vi "PSD fitting.vi"(6 "DNA length (µm)":dbl=0.658, 8 "fsampling (Hz)":dbl=2800.0, 9 "Fit settings":T2={"#PSD Averages"=40, "Correct camera acquisition artifacts"=TRUE, "Autorange"=TRUE, "fstart (Hz)"=0.0, "Pendulum geometry"=FALSE, "Fit model"=FALSE} {"#PSD Averages" min=1}, 10 "X/Y data":dbl[](array[numeric])) -> (2 "Fit Results":T1, 3 "Power spectrum (um^2/Hz)":cluster{dbl[], "Spectrum out":dbl[]}[](graph))   [LabVIEW 2017]
uses:
  <vilib>/Analysis/NI_AALPro.lvlib
  <vilib>/Analysis/NI_AALBase.lvlib
panel:
  out "df (Hz)":dbl=0.18404907975460122 format="%.2f"
  # "Fit parameters"
  # "Calculated quantities"
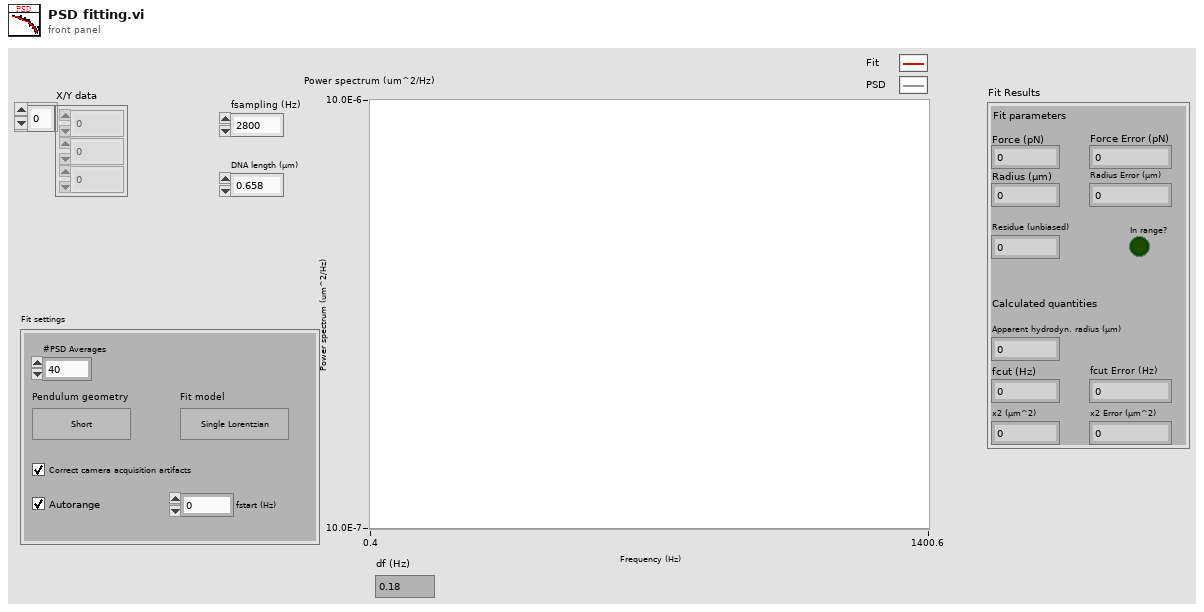
[diagram p1: front panel]
types:
  T1 = cluster{"fcut (Hz)":dbl, "x2 (µm^2)":dbl, "Force (pN)":dbl, "Radius (µm)":dbl, "Apparent hydrodyn. radius (µm)":dbl, "fcut Error (Hz)":dbl, "x2 Error (µm^2)":dbl, "Force Error (pN)":dbl, "Radius Error (µm)":dbl, "Residue (unbiased)":dbl, "In range?":bool}
  T2 = cluster{"#PSD Averages":u8, "Correct camera acquisition artifacts":bool, "Autorange":bool, "fstart (Hz)":dbl, "Pendulum geometry":bool, "Fit model":bool}
  T3 = cluster{"mean":dbl, "MSD (µm^2)":dbl, "RMS (µm)":dbl, "fc analytic (Hz)":dbl, "x2 analytic (Hz)":dbl, "RMS analytic (µm)":dbl, "F analytic (pN)":dbl, "fc fit (Hz)":dbl, "x2 fit (µm^2)":dbl, "RMS fit (µm)":dbl, "F fit (pN)":dbl, "R fit (µm)":dbl, "Rhydro (µm)":dbl, "fc Error (Hz)":dbl, "x2fit Error (µm^2)":dbl, "RMSfit Error (µm)":dbl, "Ffit Error (pN)":dbl, "Rfit Error (µm)":dbl, "correlation":dbl, "residue":dbl}
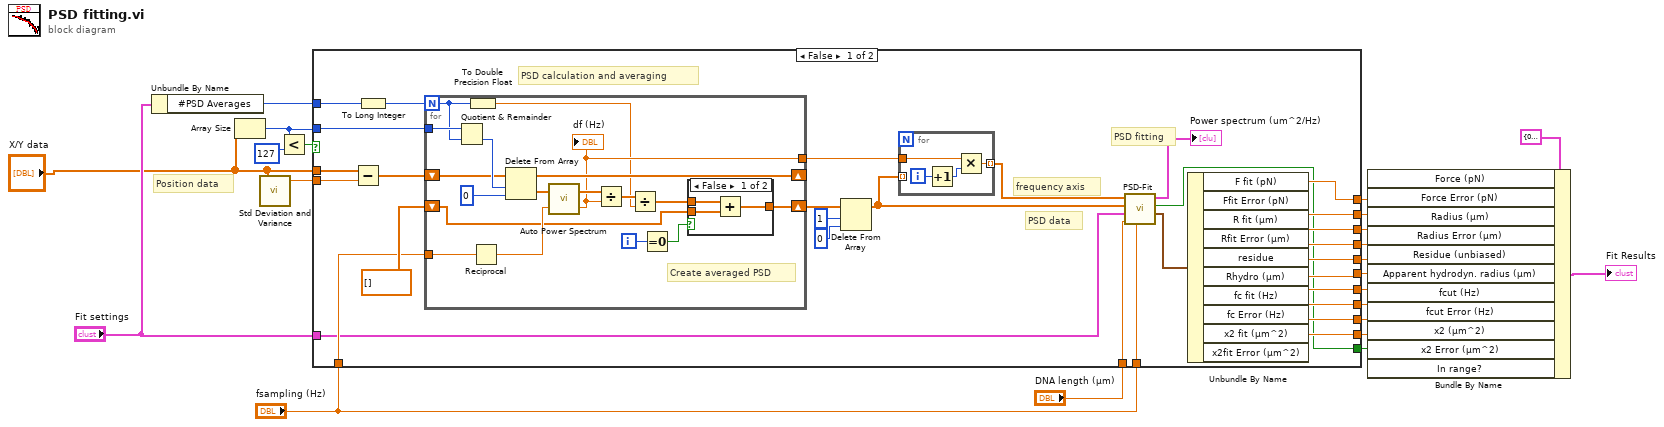
[diagram p0: block diagram]
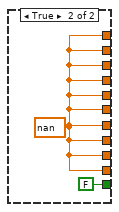
[diagram p3: hidden frame]
diagram:
  # "Position data"
  n1 = Unbundle By Name("Fit settings") -> ("#PSD Averages"=w19:u8)
  n2 = Array Size(array="X/Y data") -> (size(s)=w20:i32)
  n3 = call <vilib>:"Std Deviation and Variance.vi"("X"="X/Y data") -> ("mean"=w17:dbl)  [unwired: 1 in, 2 out]
  n4 = Less?(x=w20, y=127) -> (x < y?=w21:bool)
  n5 = case shown="False" w21 {
    tunnel: "X/Y data" -> [w50 _]
    tunnel: [w52 w80] -> w10
    tunnel: [w30 w80] -> w9
    tunnel: w20 -> [w51 _]
    tunnel: [w46 w80] -> w8
    tunnel: [w29 w80] -> w7
    tunnel: [w45 w80] -> w6
    tunnel: [w44 w80] -> w5
    tunnel: [w43 w80] -> w13
    tunnel: [w31 w80] -> w12
    tunnel: w19 -> [w38 _]
    tunnel: "Fit settings" -> [w28 _]
    tunnel: w17 -> [w34 _]
    tunnel: "fsampling (Hz)" -> [w32 _]
    tunnel: "fsampling (Hz)" -> [w27 _]
    tunnel: "DNA length (µm)" -> [w26 _]
    tunnel: [w25 w80] -> w4
    tunnel: [w24 w80] -> w3
    tunnel: [w23 FALSE ("residue in range?")] -> w2
    frame False {
      # "PSD calculation and averaging"
      # "frequency axis"
      # "PSD data"
      # "PSD fitting"
      n6 = Subtract(x=w50, y=w34) -> (x-y=w49:dbl[])
      n7 = To Long Integer(number=w38) -> (32bit integer=w47:i32)
      n8 = for {
        N: w47 -> [w65]
        tunnel: w32 -> [w69]
        tunnel: [w55] -> w37
        tunnel: w51 -> [w68]
        shift-right: [w58] -> _
        shift-left: w49 -> [w59]
        shift-right: [w64] -> w41
        shift-left: dbl[] [] ("Spectrum out") -> [w62]
        i -> [w60]
        # "Create averaged PSD"
        n9 = Quotient & Remainder(x=w68, y=w65) -> (floor(x/y)=w66:i32)  [unwired: 1 out]
        n10 = To Double Precision Float(number=w65) -> (double precision float=w53:dbl)
        n11 = Reciprocal(x=w69) -> (1/x=w70:dbl)
        n12 = Delete From Array(array=w59, length=w66, index=0) -> (deleted portion=w57:dbl[], array with subset deleted=w58:dbl[])
        n13 = call <vilib>:"Auto Power Spectrum.vi"("dt"=w70, "Signal (V)"=w57) -> ("df"=w55:dbl, "Power Spectrum (V^2 rms)"=w56:dbl[])
        "df (Hz)" <- w55
        n14 = Divide(x=w56, y=w55) -> (x/y=w54:dbl[])
        n15 = Divide(x=w54, y=w53) -> (x/y=w63:dbl[])
        n16 = Equal To 0?(x=w60) -> (x = 0?=w61:bool)
        n17 = case shown="False" w61 {
          tunnel: [w73 w74] -> w64
          tunnel: w63 -> [w72 w74]
          tunnel: w62 -> [w71 _]
          frame False {
            n18 = Add(x=w72, y=w71) -> (x+y=w73:dbl[])
          }
          frame True {
          }
        }
      }
      n19 = Delete From Array(array=w41, length=1, index=0) -> (array with subset deleted=w36:dbl[])  [unwired: 1 out]
      n20 = for {
        tunnel: w37 -> [w77]
        tunnel: [w76] -> w42 mode=indexing
        tunnel: w36 -> [_] mode=indexing
        i -> [w78]
        n21 = Increment(x=w78) -> (x+1=w75:i32)
        n22 = Multiply(x=w77, y=w75) -> (x*y=w76:dbl)
      }
      n23 = call "PSD-Fit.vi"("fsampling (Hz)"=w27, "DNA length (µm)"=w26, "Fit settings"=w28, "PSD (um^2/Hz)"=w36, "f (Hz)"=w42) -> ("Fit Results"=w33:T3, "residue in range?"=w23:bool, "Power spectrum (um^2/Hz)"=→"Power spectrum (um^2/Hz)":cluster{dbl[], "Spectrum out":dbl[]}[])  [unwired: 1 out]
      n24 = Unbundle By Name(w33) -> ("F fit (pN)"=w43:dbl, "Ffit Error (pN)"=w31:dbl, "R fit (µm)"=w52:dbl, "Rfit Error (µm)"=w30:dbl, "residue"=w46:dbl, "Rhydro (µm)"=w29:dbl, "fc fit (Hz)"=w45:dbl, "fc Error (Hz)"=w44:dbl, "x2 fit (µm^2)"=w25:dbl, "x2fit Error (µm^2)"=w24:dbl)
    }
    frame True {
      (unwired) FALSE ("residue in range?")
      (unwired) dbl[][] [[nan]]
      w80 = nan
    }
  }
  n25 = Bundle By Name(cluster=T1 {"fcut (Hz)"=0.0, "x2 (µm^2)"=0.0, "Force (pN)"=0.0, "Radius (µm)"=0.0, "Apparent hydrodyn. radius (µm)"=0.0, "fcut Error (Hz)"=0.0, "x2 Error (µm^2)"=0.0, "Force Error (pN)"=0.0, "Radius Error (µm)"=0.0, "Residue (unbiased)"=0.0, "In range?"=FALSE} ("Fit Results 3"), "Force (pN)"=w13, "Force Error (pN)"=w12, "Radius (µm)"=w10, "Radius Error (µm)"=w9, "Residue (unbiased)"=w8, "Apparent hydrodyn. radius (µm)"=w7, "fcut (Hz)"=w6, "fcut Error (Hz)"=w5, "x2 (µm^2)"=w4, "x2 Error (µm^2)"=w3, "In range?"=w2) -> (→"Fit Results":T1)
